vi "sample obtain bucket put object.vi"() -> ()   [LabVIEW 2015]
uses:
  GET Object Result Parameters.ctl
  Core/HTTP Request/AWS Credentials.ctl
  PUT Object Request Parameters.ctl
  ACL.ctl
  Storage Class.ctl
  Core/HTTP Request/Name Value Pair.ctl
  GET Object Request Parameters.ctl
  Core/Request Range.ctl
  Bucket/Bucket.lvclass
  Core/HTTP Request/HTTP Request.lvclass
  NI_AWS_S3.lvlib
  Core/NI_AWS_Core.lvlib
panel:
  out "GetObjectResult":T1
  out "Object Data":string
  out "error out":errorcluster
  in  "Bucket name":string="bpreis-test-95"
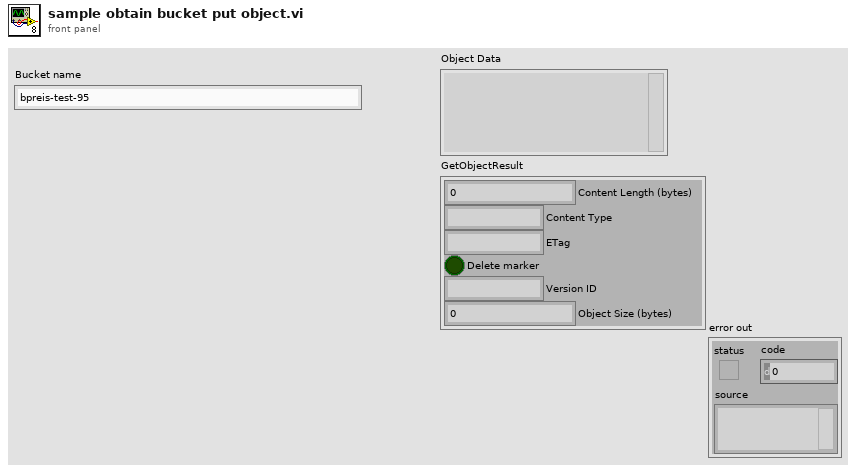
[diagram p1: front panel]
types:
  T1 = typedef "NI_AWS_S3.lvlib/GET Object Result Parameters.ctl" = cluster{"Content Length (bytes)":u64, "Content Type":string, "ETag":string, "Delete marker":bool, "Version ID":string, "Object Size (bytes)":u64}
  T2 = typedef "NI_AWS_S3.lvlib/GET Object Request Parameters.ctl" = cluster{"Range":T3, "If Modified Since":timestamp, "If Unmodified Since":timestamp, "Matching ETag":string, "Nonmatching ETag":string}
  T3 = typedef "NI_AWS_Core.lvlib/Request Range.ctl" = cluster{"Start":i64, "Length":i64}
  T4 = typedef "NI_AWS_S3.lvlib/PUT Object Request Parameters.ctl" = cluster{"Content Type":string, "ACL":T5, "Storage Class":T6, "User Metadata":T7[], "Content MD5":string}
  T5 = typedef "NI_AWS_S3.lvlib/ACL.ctl" = enum16{"private", "public-read", "public-read-write", "aws-exec-read", "authenticated-read", "bucket-owner-read", "bucket-owner-full-control"}
  T6 = typedef "NI_AWS_S3.lvlib/Storage Class.ctl" = enum16{"STANDARD", "REDUCED_REDUNDANCY"}
  T7 = typedef "NI_AWS_Core.lvlib/HTTP Request.lvclass/Name Value Pair.ctl" = cluster{"name":string, "value":string}
  T8 = typedef "NI_AWS_Core.lvlib/HTTP Request.lvclass/AWS Credentials.ctl" = cluster{"Access Key":string, "Secret Key":string}
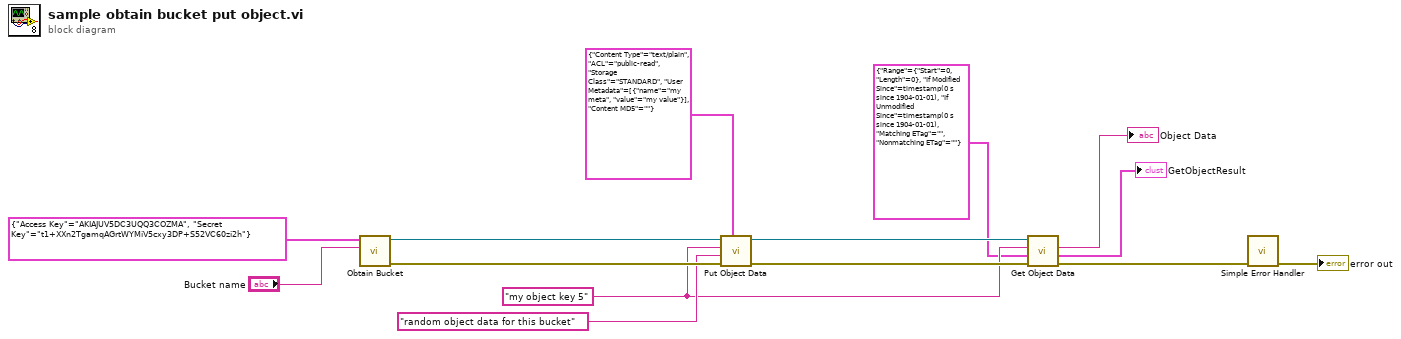
[diagram p0: block diagram]
diagram:
  w4 = "my object key 5" ("Object Key")
  n1 = call "Obtain Bucket.vi"("Bucket name"="Bucket name", "AWS Credentials"=T8 {"Access Key"="AKIAJUV5DC3UQQ3COZMA", "Secret Key"="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"}) -> ("error out"=w14:errorcluster, "Bucket"=w10:refnum<class "Bucket.lvclass">)  [unwired: 8 in]
  n2 = call "Put Object Data.vi"("PUT Object Request Parameters"=T4 {"Content Type"="text/plain", "ACL"=enum."public-read", "Storage Class"=enum."STANDARD", "User Metadata"=[{"name"="my meta", "value"="my value"}], "Content MD5"=""}, "error in (no error)"=w14, "Object Data"="random object data for this bucket", "Object Key"=w4, "Bucket in"=w10) -> ("error out"=w7:errorcluster, "Bucket out"=w5:refnum<class "Bucket.lvclass">)  [unwired: 5 in]
  n3 = call "Get Object Data.vi"("error in (no error)"=w7, "Request Parameters"=T2 {"Range"={"Start"=0, "Length"=0}, "If Modified Since"=timestamp(0 s since 1904-01-01), "If Unmodified Since"=timestamp(0 s since 1904-01-01), "Matching ETag"="", "Nonmatching ETag"=""}, "Object Key"=w4, "Bucket in"=w5) -> ("error out"=w6:errorcluster, "GetObjectResult"=→"GetObjectResult":T1, "Object Data"=→"Object Data":string)  [unwired: 4 in, 1 out]
  n4 = call <vilib>:"Simple Error Handler.vi"("error in (no error)"=w6) -> ("error out"=→"error out":errorcluster)  [unwired: 4 in, 4 out]
